vi "Get DBL Array from Str.vi"(11 "String":string="1E-6; 2,5E-6; 5E-6; 7,5E-6") -> (2 "Array":dbl[](array[numeric]))   [LabVIEW 2018]
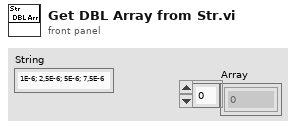
[diagram p1: front panel]
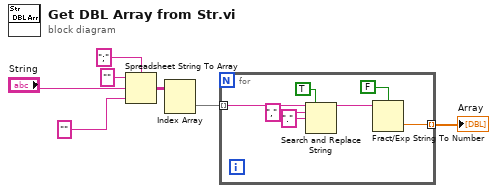
[diagram p0: block diagram]
diagram:
  n1 = Spreadsheet String To Array(delimiter (Tab)=";", format string="", spreadsheet string="String", array type (2D Dbl)="" ("format string")) -> (array=w5:string[][])
  n2 = Index Array(array=w5) -> (element=w2:string[])  [unwired: 2 in]
  n3 = for {
    tunnel: w2 -> [w12] mode=indexing
    tunnel: [w14] -> w1 mode=indexing
    n4 = Search and Replace String(replace all?=TRUE ("replace all? (F)"), input string=w12, search string=",", replace string="." ("replace string (\"\")")) -> (result string=w9:string)  [unwired: 4 in, 3 out]
    n5 = Fract/Exp String To Number(use system decimal point (T)=FALSE, string=w9) -> (number=w14:dbl)  [unwired: 2 in, 1 out]
  }
  "Array" <- w1
